vi "Present.vi"(8 "error in (no error)":errorcluster, 11 "Renderer":refnum<class "Renderer.lvclass">) -> (0 "error out":errorcluster)   [LabVIEW 2021, in "Renderer.lvclass"]
uses:
  Renderer.lvclass
  Renderer.lvclass/Renderer.ctl
  LabSDL2/Source/Libraries/LibSDL2 Wrapper/LibSDL2.lvlib
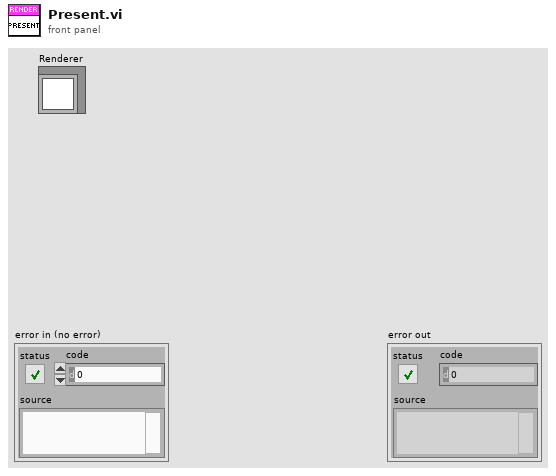
[diagram p1: front panel]
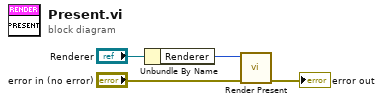
[diagram p0: block diagram]
diagram:
  n1 = Unbundle By Name("Renderer") -> ("Renderer"=w4:u32)
  n2 = call "Render Present.vi"("error in"="error in (no error)", "Renderer Pointer"=w4) -> ("error out"=→"error out":errorcluster)  [unwired: 9 in]
